vi "GOOPDebugger_AddDebugging.vi"(7 "Action":T1=enum."GeneratePattern", 8 "error in (no error)":errorcluster, 10 "DataIn":variant, 11 "ClassRefToActOn":refnum<vi>) -> (0 "error out":errorcluster, 1 "Name":string, 2 "DataOut":variant, 3 "Cancelled":bool)   [LabVIEW 2020]
uses:
  <resource>/Framework/Providers/Open_GDS/ClassProviders/Provider_BaseClassInterface/BaseProvider_SubVIs/BaseProvider_DesignPatternsActions.ctl
  <resource>/Framework/Providers/Open_GDS/ClassProviders/Common/LvClass_class/GDSLvClass_ProviderTypes.ctl
  <resource>/Framework/Providers/Open_GDS/ClassProviders/Provider_EndevoGOOP400/EndevoG4ProviderName.ctl
  <vilib>/picture/picture.llb/imagedata.ctl
panel:
  in  "_Cancel":bool
  in  "_OK":bool
  # "Debugging"
  # "This option will add debugging functions to the class"
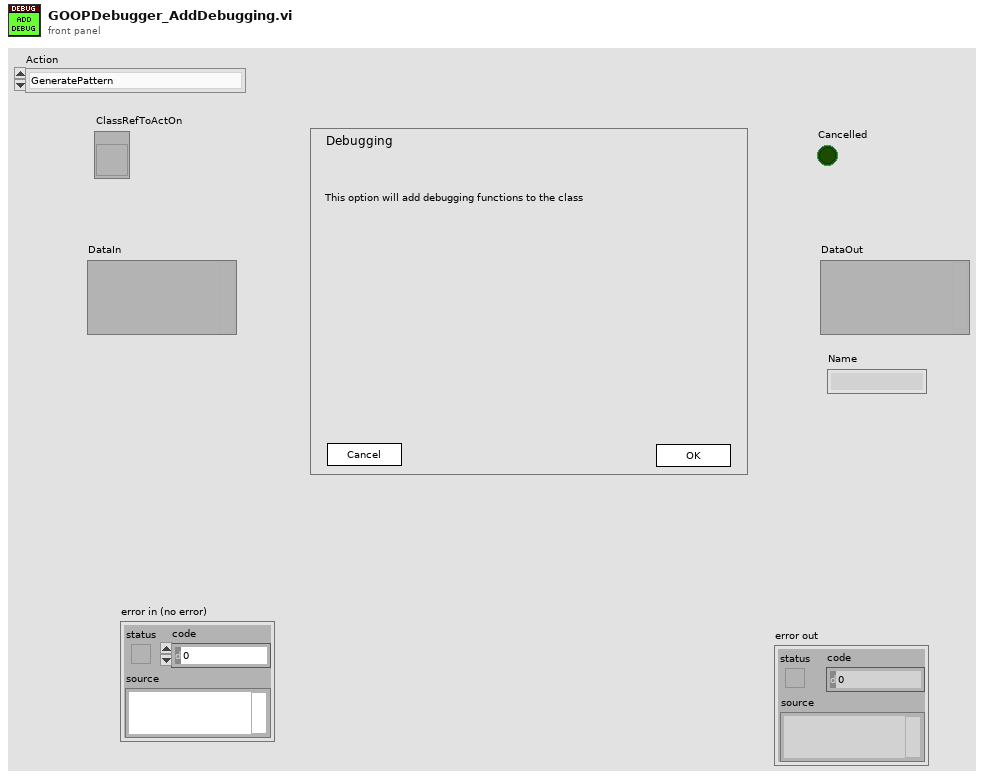
[diagram p1: front panel]
types:
  T1 = typedef "BaseProvider_DesignPatternsActions.ctl" = enum16{"AddPatternDialog", "GeneratePattern", "RemovePattern", "CreatePatternMethod", "UpdatePattern"}
  T2 = typedef "GDSLvClass_ProviderTypes.ctl" = enum16{"UnKnown(LabVOOP)", "Native", "EndevoGOOP3", "OpenG(RootObject)", "OpenG(OpenG_Object)", "EndevoGOOP4", "JKI1"}
  T3 = cluster{"Application":refnum<vi>, "SupportFolder":path, "TemplateName":string, "ClassProvider":T2, "UtilsFolder":path, "UtilsFolderRef":refnum<vi>, "ClassName":string, "Template_GetObjectStatus":path, "ProcessIdRef":refnum<vi>, "Template_GetObjectStatusRef":refnum<vi>, "ProtectedFolder":path, "ClassAttribute":bool}
  T4 = cluster{"Cancelled":bool, "Files":path[], "ClassPath":path, "DataOut":variant}
  T5 = typedef "EndevoG4ProviderName.ctl" = enum16{"EndevoGOOP400"}
  T6 = enum32{"invalid lock state", "Not Locked", "Locked (No Password)", "Password-protected"}
  T7 = typedef "imagedata.ctl" = cluster{"image type":i32, "image depth":i32, "image":u8[], "mask":u8[], "colors":u32[], "Rectangle":cluster{"left":i16, "top":i16, "right":i16, "bottom":i16}}
  T8 = typedef "GDSLvCLass_ClassSettingsType.ctl" = cluster{"ClassProviderName":string, "ClassTemplateUsed":string, "ClassTemplateVersion":string, "ClassDescription":string, "PlugIns":T9[], "ConnectorPanePattern":string}
  T9 = typedef "GDSLvClass_PlugIn.ctl" = cluster{"Type":T10, "ID":string, "Version":string, "Path":path, "Name":string, "Data":variant}
  T10 = typedef "GDSLvClass_PlugInTypes.ctl" = enum16{"DesignPattern", "MethodTypes"}
  T11 = typedef "GOOP400_Options.ctl" = cluster{"FlatFolderStructure":bool}
  T12 = typedef "GDSLvClass_IconSettingsType.ctl" = cluster{"Frame":u32, "Frame thickness":u8, "Header Background":u32, "Header Text":u32, "ColorPublic":u32, "ColorProtected":u32, "ColorPrivate":u32, "Body Text":u32, "ClassBodyIcon":string}
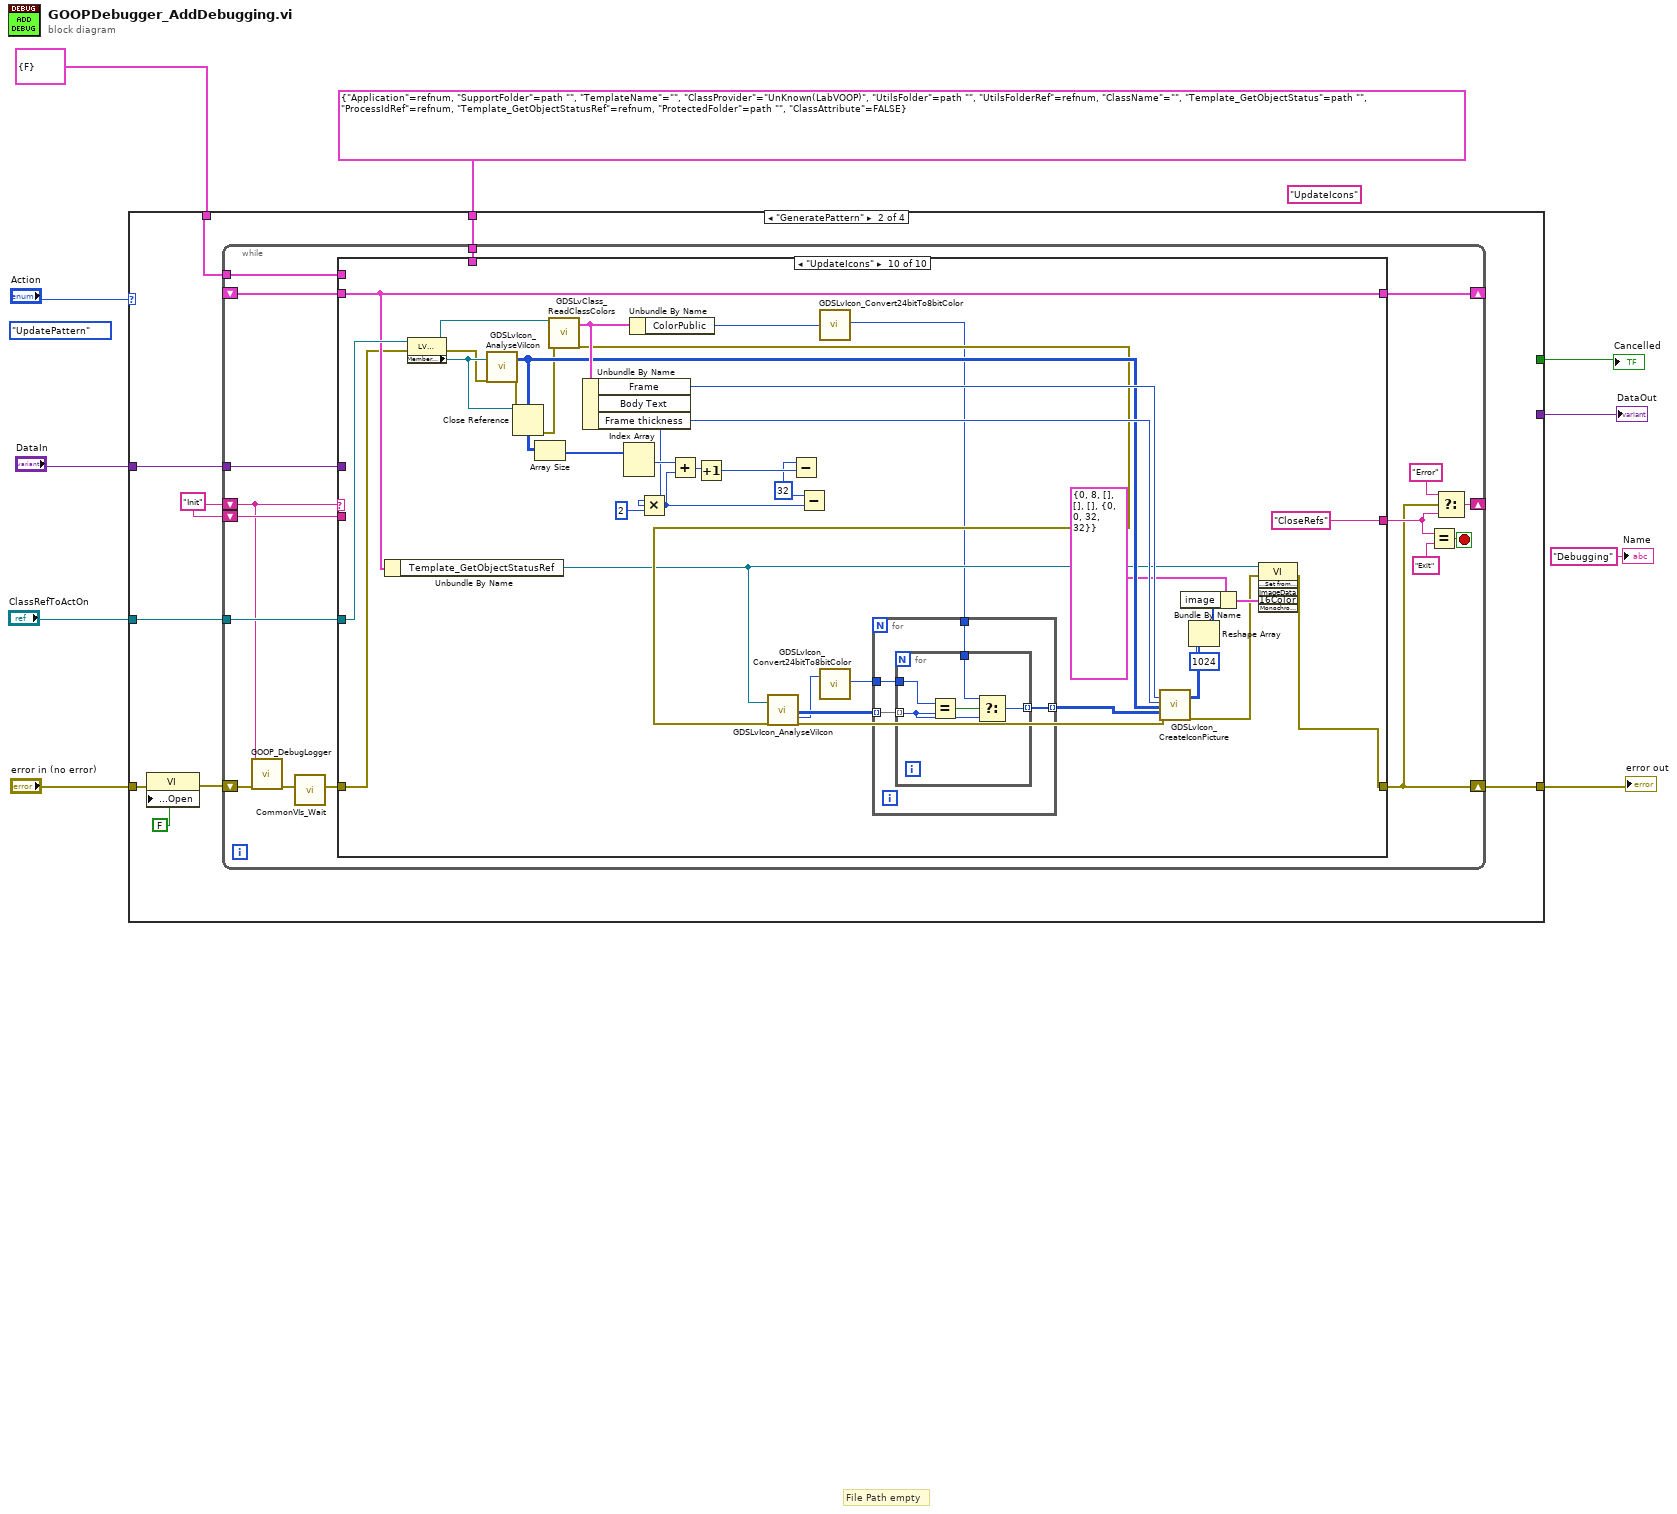
[diagram p0: block diagram]
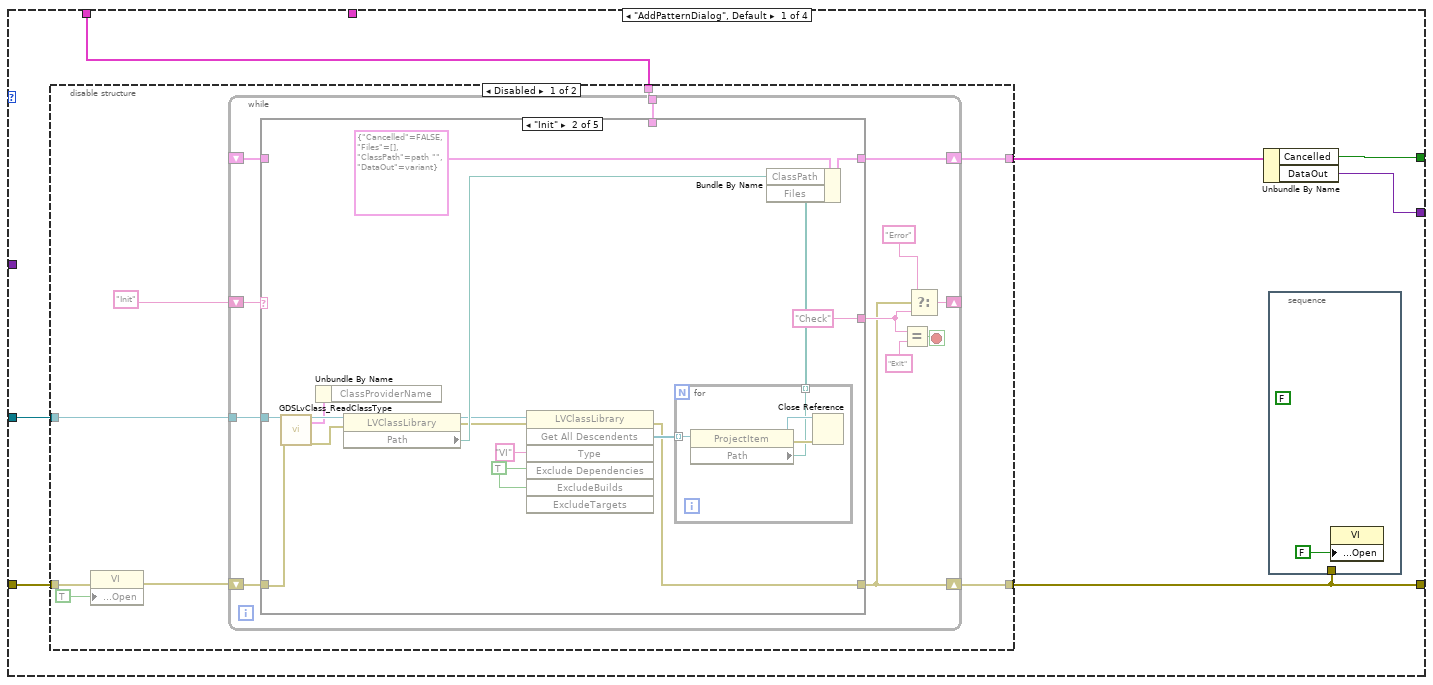
[diagram p2: hidden frame]
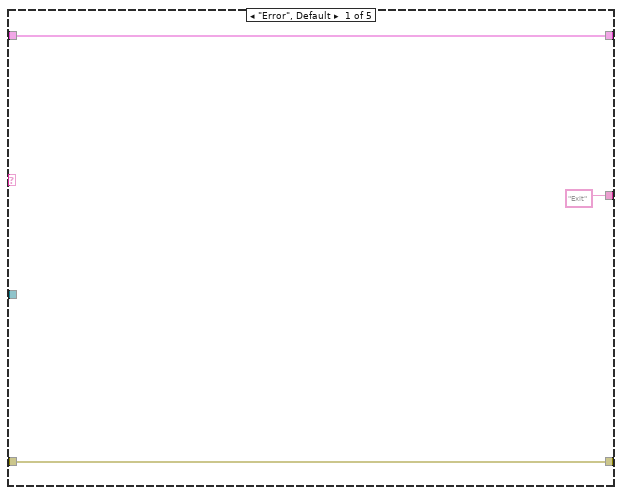
[diagram p3: hidden frame]
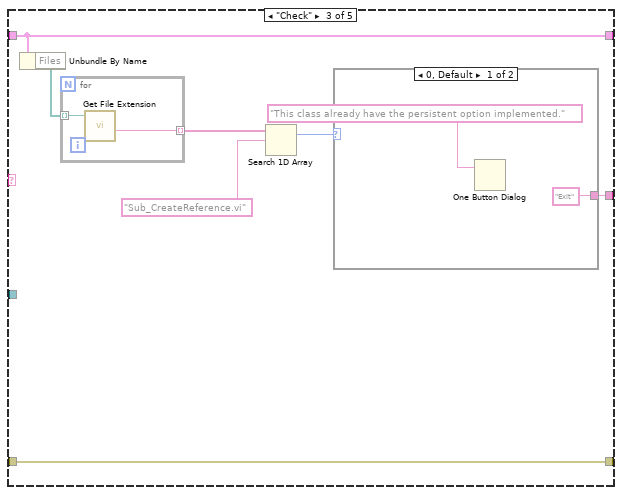
[diagram p4: hidden frame]
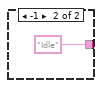
[diagram p5: hidden frame]
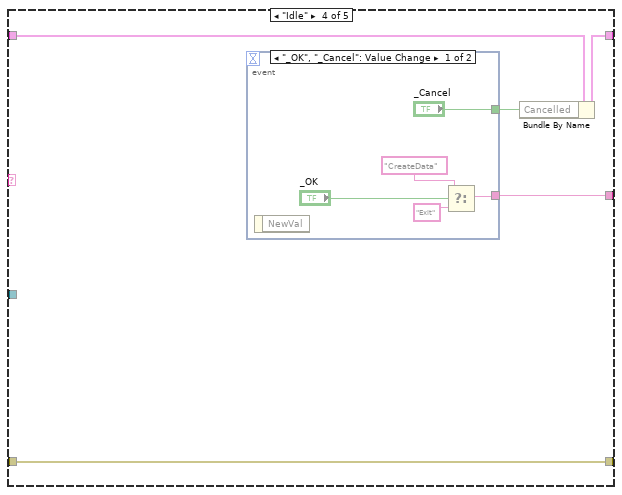
[diagram p6: hidden frame]
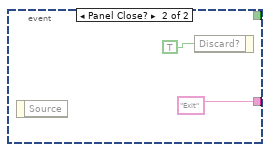
[diagram p7: hidden frame]
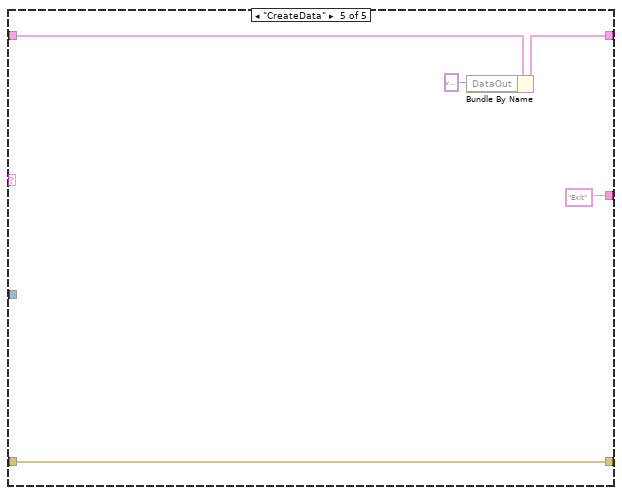
[diagram p8: hidden frame]
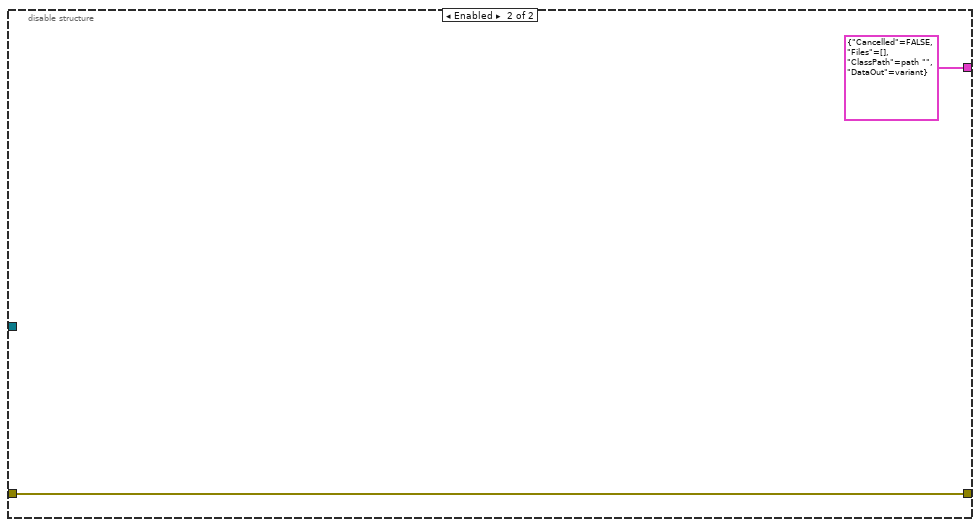
[diagram p9: hidden frame]
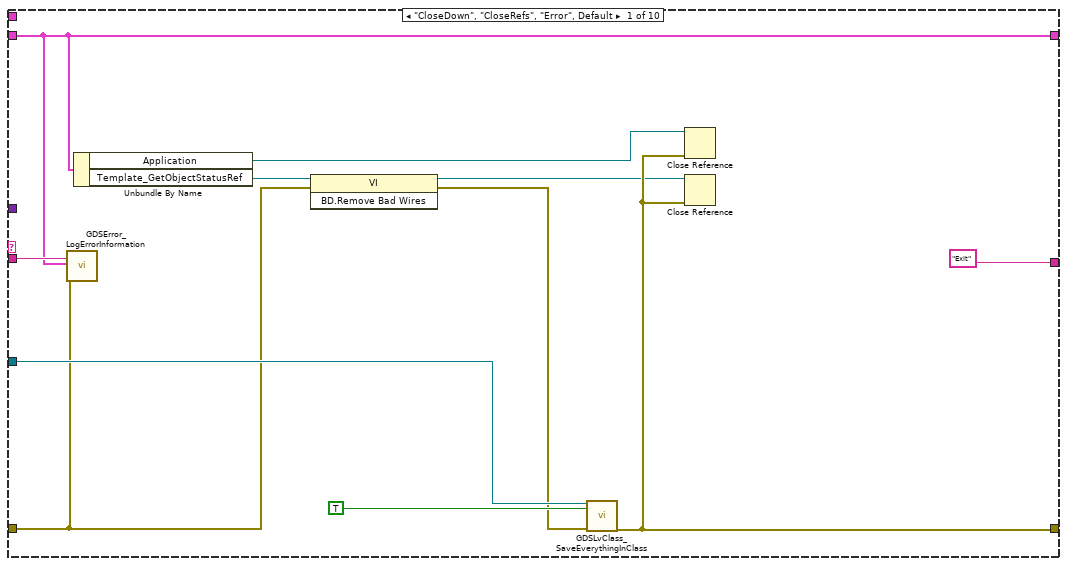
[diagram p10: hidden frame]
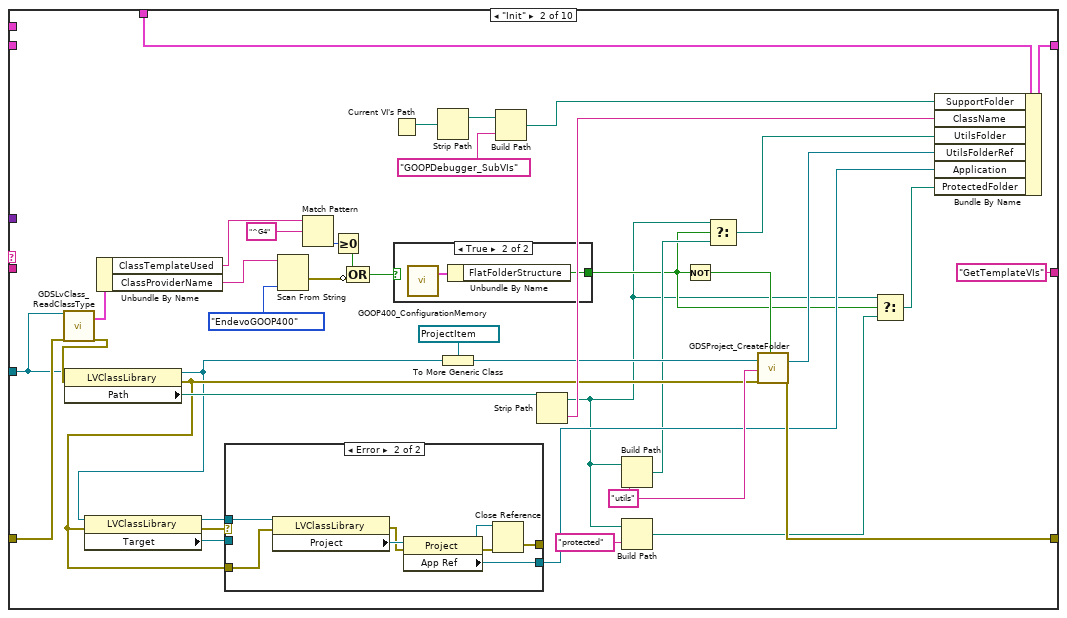
[diagram p11: hidden frame]
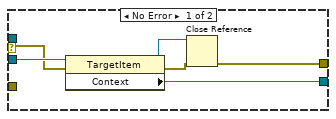
[diagram p13: hidden frame]
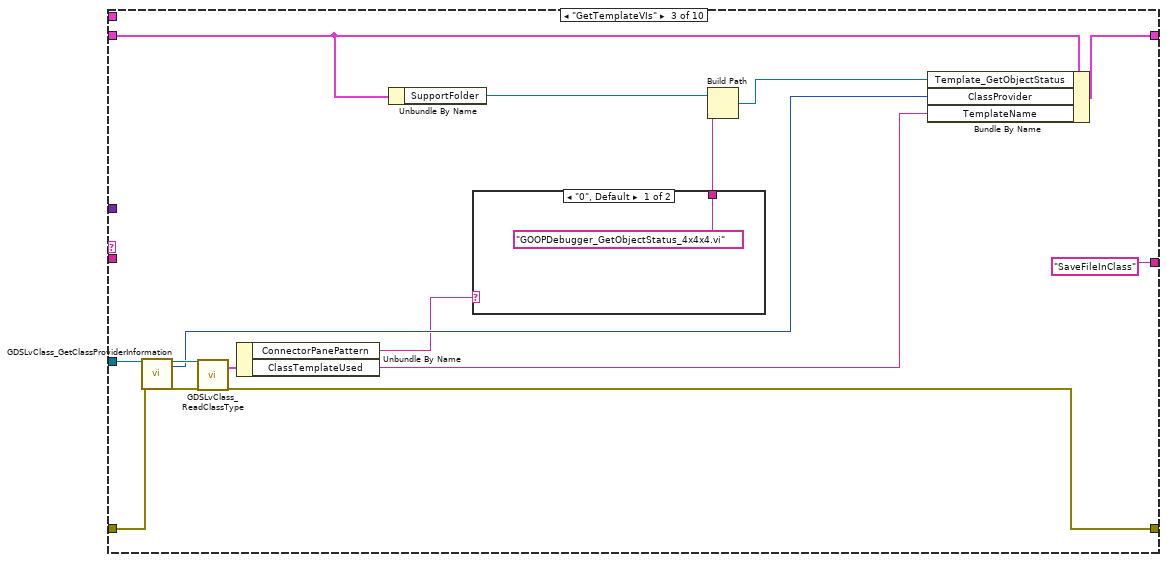
[diagram p14: hidden frame]
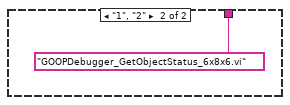
[diagram p15: hidden frame]
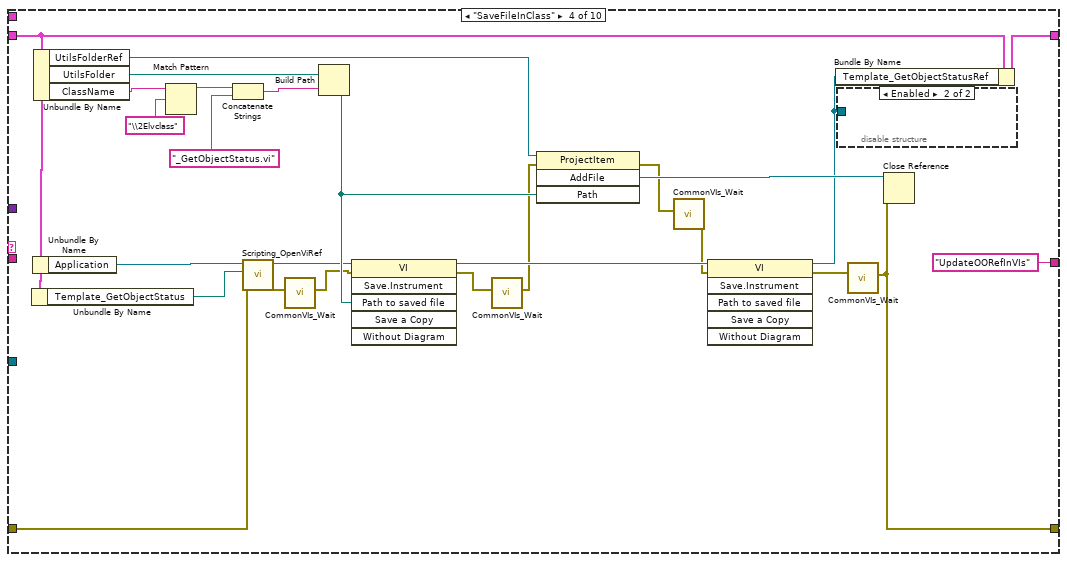
[diagram p16: hidden frame]
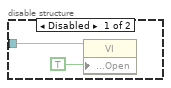
[diagram p17: hidden frame]
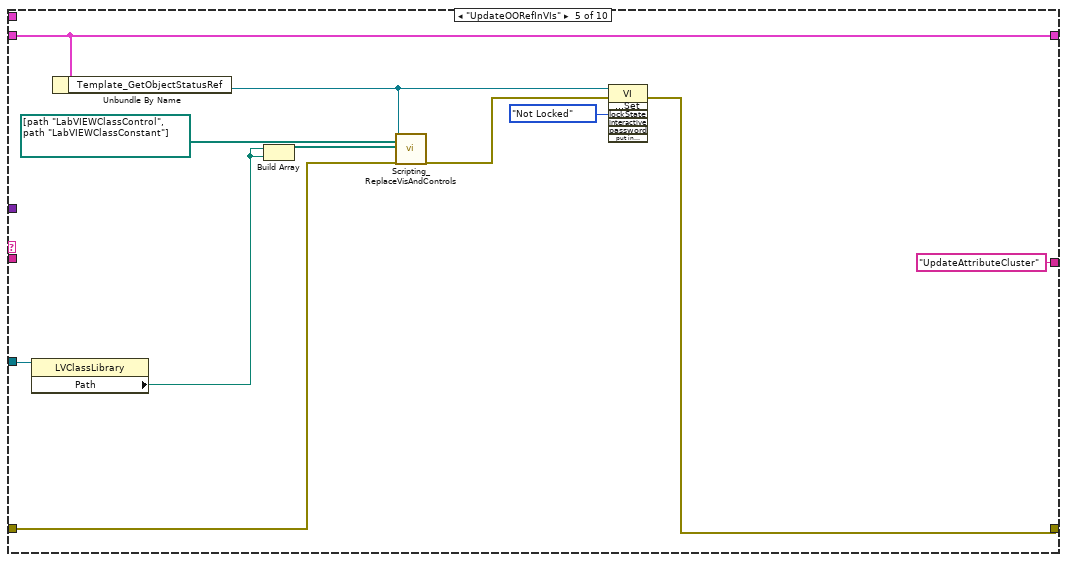
[diagram p18: hidden frame]
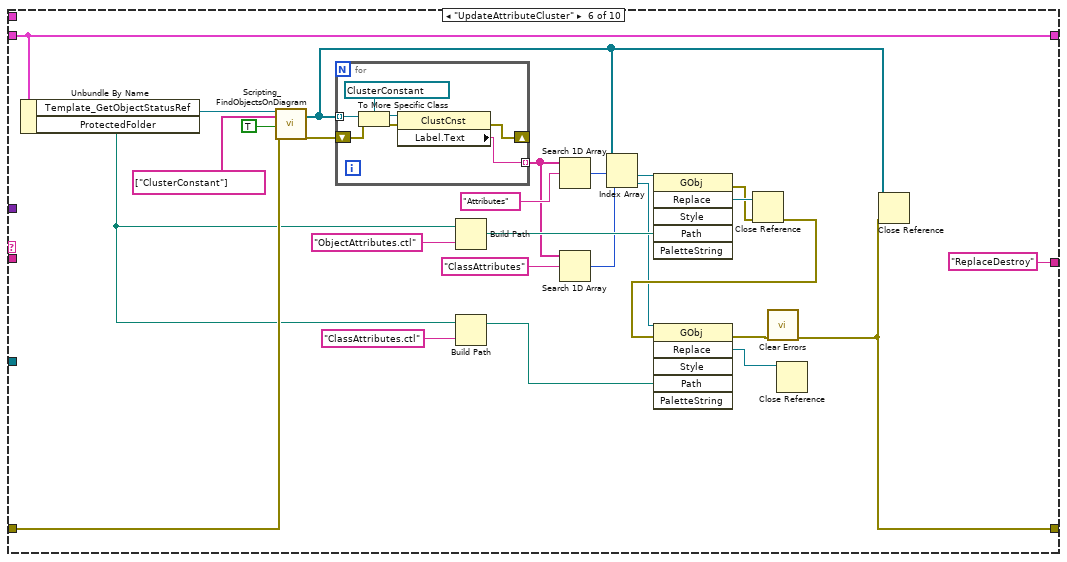
[diagram p19: hidden frame]
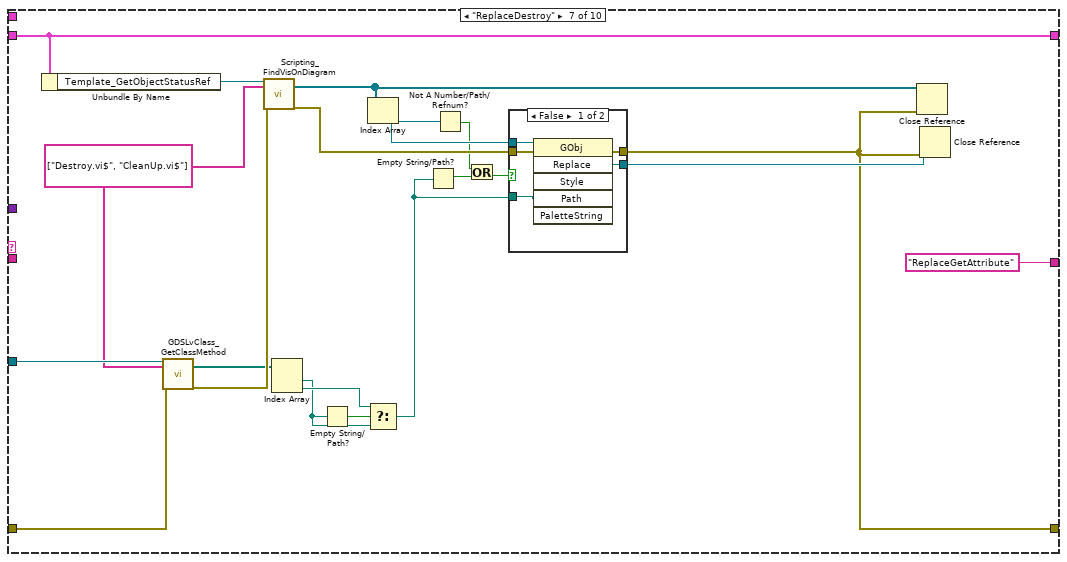
[diagram p20: hidden frame]
diagram:
  (unwired) "UpdateIcons"
  (unwired) BaseProvider_DesignPatternsActions."UpdatePattern" ("Action")
  # "File Path empty"
  n1 = case shown="\"GeneratePattern\"" "Action" {
    tunnel: "error in (no error)" -> [w17 w95 w421 w422]
    tunnel: [w16 w101 w421 w422] -> w8
    tunnel: "ClassRefToActOn" -> [w14 w97 _ _]
    tunnel: [w13 _ _ _] -> w6
    tunnel: [w12 _ _ _] -> w5
    tunnel: cluster{"Settings":bool} {"Settings"=FALSE} ("output cluster") -> [w11 w99 _ _]
    tunnel: "DataIn" -> [_ w100 _ _]
    tunnel: T3 {"Application"=refnum, "SupportFolder"=path "", "TemplateName"="", "ClassProvider"=enum."UnKnown(LabVOOP)", "UtilsFolder"=path "", "UtilsFolderRef"=refnum, "ClassName"="", "Template_GetObjectStatus"=path "", "ProcessIdRef"=refnum, "Template_GetObjectStatusRef"=refnum, "ProtectedFolder"=path "", "ClassAttribute"=FALSE} -> [_ w98 _ _]
    frame "AddPatternDialog", Default {
      n2 = disable-structure shown="Disabled" {
        disable-tunnel: w17 -> [w24 w91]
        disable-tunnel: [w21 w91] -> w16
        disable-tunnel: [w20 T4 {"Cancelled"=FALSE, "Files"=[], "ClassPath"=path "", "DataOut"=variant}] -> w15
        disable-tunnel: w14 -> [w19 _]
        disable-tunnel: w11 -> [w18 _]
        frame Disabled {
          n3 = property class="VI"(error in=w24, "Front Panel.Open"=TRUE ("Front Panel Window:Open")) -> (error out=w23:errorcluster)  [unwired: 1 in, 1 out]
          n4 = while {
            shift-right: [w30] -> w21
            shift-left: w23 -> [w37]
            shift-right: [w35] -> _
            shift-left: "Init" -> [w36]
            shift-right: [w29] -> w20
            shift-left: _ -> [w28]
            tunnel: w19 -> [w27]
            tunnel: w18 -> [w26]
            stop <- w34 stop-if-true
            n5 = case shown="\"Init\"" w36 {
              tunnel: w37 -> [w40 w43 w64 w76 w86]
              tunnel: [w40 w52 w64 w76 w86] -> w30
              tunnel: ["Exit" "Check" w66 w77 "Exit"] -> w31
              tunnel: [w38 w50 w65 w75 w88] -> w29
              tunnel: w28 -> [w38 _ w65 w73 w89]
              tunnel: w27 -> [_ w45 _ _ _]
              tunnel: w26 -> [_ _ _ _ _]
              frame "Error", Default {
              }
              frame "Init" {
                w54 = TRUE ("ExcludeDependencies")
                n6 = call <resource>:"GDSLvClass_ReadClassType.vi"("Class Refnum In"=w45, "error in (no error)"=w43) -> ("Class Refnum Out"=w44:refnum<vi>, "ClassSettings"=w41:T8, "error out"=w42:errorcluster)  [unwired: 15 in]
                n7 = Unbundle By Name(w41) -> ()  [unwired: 1 out]
                n8 = property class="LVClassLibrary"(reference=w44, error in=w42) -> (reference out=w47:refnum<vi>, error out=w46:errorcluster, "Path"=w49:path)
                n9 = invoke class="LVClassLibrary" method="Get All Descendents"(reference=w47, error in=w46, "Type"="VI", "Exclude Dependencies"=w54, "ExcludeBuilds"=w54) -> (error out=w52:errorcluster, "All Descendents"=w53:refnum<vi>[])  [unwired: 2 in, 5 out]
                n10 = for {
                  tunnel: w53 -> [w60] mode=indexing
                  tunnel: [w57] -> w48 mode=indexing
                  n11 = property class="ProjectItem"(reference=w60) -> (reference out=w58:refnum<vi>, error out=w59:errorcluster, "Path"=w57:path)  [unwired: 1 in]
                  n12 = Close Reference(reference=w58, error in (no error)=w59) -> ()  [unwired: 1 out]
                }
                n13 = Bundle By Name(cluster=T4 {"Cancelled"=FALSE, "Files"=[], "ClassPath"=path "", "DataOut"=variant}, "ClassPath"=w49, "Files"=w48) -> (w50:T4)
              }
              frame "Check" {
                n14 = Unbundle By Name(w65) -> ("Files"=w67:path[])
                n15 = for {
                  tunnel: w67 -> [w72] mode=indexing
                  tunnel: [w71] -> w63 mode=indexing
                  n16 = call <vilib>:"Get File Extension.vi"("file"=w72) -> ("filename without extension"=w71:string)  [unwired: 6 in, 4 out]
                }
                n17 = Search 1D Array(1D array=w63, element="Sub_CreateReference.vi") -> (index of element=w61:i32)  [unwired: 1 in]
                n18 = case shown="0, Default" w61 {
                  tunnel: ["Exit" "Idle"] -> w66
                  frame 0, Default {
                    n19 = One Button Dialog(message="This class already have the persistent option implemented.") -> ()  [unwired: 1 in, 1 out]
                  }
                  frame -1 {
                  }
                }
              }
              frame "Idle" {
                n20 = event shown="[0] \"_OK\", \"_Cancel\": Value Change" {
                  selector: _ -> [_ _]
                  dyn-events: _ -> [_ _]
                  timeout: _ -> [_ _]
                  tunnel: [w81 "Exit"] -> w77
                  tunnel: ["_Cancel" _] -> w74
                  event "_OK", "_Cancel": Value Change {
                    n21 = event-data() -> ()  [unwired: 1 in, 1 out]
                    n22 = Select(t="CreateData", s="_OK", f="Exit") -> (s? t:f=w81:string)
                  }
                  event Panel Close? {
                    n23 = event-data() -> ()  [unwired: 1 in, 1 out]
                    n24 = event-data("Discard?"=TRUE) -> ()  [unwired: 1 in, 1 out]
                  }
                }
                n25 = Bundle By Name(cluster=w73, "Cancelled"=w74) -> (w75:T4)
              }
              frame "CreateData" {
                n26 = Bundle By Name(cluster=w89, "DataOut"=variant) -> (w88:T4)
              }
            }
            n27 = Equal?(x=w31, y="Exit") -> (x = y?=w34:bool)
            n28 = Select(t="Error", s=w30, f=w31) -> (s? t:f=w35:string)
          }
        }
        frame Enabled {
        }
      }
      n29 = Unbundle By Name(w15) -> ("Cancelled"=w13:bool, "DataOut"=w12:variant)
      n30 = stacked-sequence {
        tunnel: w16 -> [_]
        frame #0 {
          (unwired) FALSE ("Visible")
          n31 = property class="VI"("Front Panel.Open"=FALSE ("Front Panel Window:Open")) -> ()  [unwired: 2 in, 2 out]
        }
      }
    }
    frame "GeneratePattern" {
      w93 = "Init"
      n32 = property class="VI"(error in=w95, "Front Panel.Open"=FALSE ("Front Panel Window:Open")) -> (error out=w94:errorcluster)  [unwired: 1 in, 1 out]
      n33 = while {
        shift-right: [w113] -> w101
        shift-left: w94 -> [w105]
        shift-right: [w118] -> _
        shift-left: w93 -> [w104]
        shift-right: [w112] -> _
        shift-left: _ -> [w111]
        tunnel: w100 -> [w110]
        tunnel: w99 -> [w109]
        tunnel: w98 -> [w108]
        tunnel: w97 -> [w107]
        shift-left: w93 -> [w106]
        stop <- w117 stop-if-true
        n34 = call <resource>:"GOOP_DebugLogger.vi"("error in (no error)"=w105, "State"=w104) -> ("error out"=w103:errorcluster)  [unwired: 7 in, 2 out]
        n35 = call <resource>:"CommonVIs_Wait.vi"("error in"=w103) -> ("error out"=w102:errorcluster)  [unwired: 9 in]
        n36 = case shown="\"UpdateIcons\"" w104 {
          tunnel: w102 -> [w120 w139 w199 w222 w240 w257 w288 w321 w362 w391]
          tunnel: [w125 w161 w188 w203 w234 w245 w275 w322 w361 w390] -> w113
          tunnel: ["Exit" "GetTemplateVIs" "SaveFileInClass" "UpdateOORefInVIs" "UpdateAttributeCluster" "ReplaceDestroy" "ReplaceGetAttribute" w311 "UpdateIcons" "CloseRefs"] -> w114
          tunnel: [w123 w168 w198 w228 w241 w242 w285 w309 w360 w393] -> w112
          tunnel: w111 -> [w123 _ w193 w226 w241 w242 w285 w310 w360 w393]
          tunnel: w110 -> [_ _ _ _ _ _ _ _ _ _]
          tunnel: w109 -> [_ _ _ _ _ _ _ _ _ _]
          tunnel: w108 -> [_ w167 _ _ _ _ _ _ _ _]
          tunnel: w107 -> [w127 w138 w200 _ w239 _ w290 w318 _ w394]
          tunnel: w106 -> [w124 _ _ _ _ _ _ _ _ _]
          frame "CloseDown", "CloseRefs", "Error", Default {
            n37 = call <resource>:"GDSError_LogErrorInformation.vi"("State"=w124, "LocalVariableData"=w123, "error in (no error)"=w120) -> ()  [unwired: 16 in, 1 out]
            n38 = Unbundle By Name(w123) -> ("Application"=w126:refnum<vi>, "Template_GetObjectStatusRef"=w122:refnum<vi>)
            n39 = invoke class="VI" method="BD.Remove Bad Wires"(reference=w122, error in=w120) -> (reference out=w121:refnum<vi>, error out=w119:errorcluster)  [unwired: 1 in, 1 out]
            n40 = call <resource>:"GDSLvClass_SaveEverythingInClass.vi"("ClassRefIn"=w127, "ForceResaving(False)"=TRUE, "error in"=w119) -> ("error out"=w125:errorcluster)  [unwired: 15 in, 1 out]
            n41 = Close Reference(reference=w126, error in (no error)=w125) -> ()  [unwired: 1 out]
            n42 = Close Reference(reference=w121, error in (no error)=w125) -> ()  [unwired: 1 out]
          }
          frame "Init" {
            w157 = "utils" ("name or relative path")
            n43 = call <resource>:"GDSLvClass_ReadClassType.vi"("Class Refnum In"=w138, "error in (no error)"=w139) -> ("ClassSettings"=w143:T8, "error out"=w140:errorcluster)  [unwired: 15 in, 1 out]
            n44 = property class="LVClassLibrary"(reference=w138, error in=w140) -> (reference out=w130:refnum<vi>, error out=w150:errorcluster, "Path"=w162:path)
            n45 = property class="LVClassLibrary"(reference=w130, error in=w150) -> (reference out=w152:refnum<vi>, error out=w154:errorcluster, "Target"=w153:refnum<vi>)
            n46 = Unbundle By Name(w143) -> ("ClassTemplateUsed"=w142:string, "ClassProviderName"=w141:string)
            n47 = case shown="Error" w154 {
              selector: w154 -> [w173 _]
              tunnel: w153 -> [w177 _]
              tunnel: [w176 w179] -> w151
              tunnel: [w172 w180] -> _
              tunnel: w152 -> [_ w185]
              tunnel: w150 -> [_ w184]
              frame No Error {
                n48 = property class="TargetItem"(reference=w177, error in=w173) -> (reference out=w174:refnum<vi>, error out=w175:errorcluster, "Context"=w176:refnum<vi>)
                n49 = Close Reference(reference=w174, error in (no error)=w175) -> (error out=w172:errorcluster)
              }
              frame Error {
                n50 = property class="LVClassLibrary"(reference=w185, error in=w184) -> (error out=w178:errorcluster, "Project"=w183:refnum<vi>)  [unwired: 1 out]
                n51 = property class="Project"(reference=w183, error in=w178) -> (reference out=w181:refnum<vi>, error out=w182:errorcluster, "App Ref"=w179:refnum<vi>)
                n52 = Close Reference(reference=w181, error in (no error)=w182) -> (error out=w180:errorcluster)
              }
            }
            n53 = Scan From String(input string=w141, default 1=EndevoG4ProviderName."EndevoGOOP400" ("ProviderName")) -> (error out=w147:errorcluster)  [unwired: 4 in, 2 out]
            n54 = Match Pattern(string=w142, regular expression="^G4") -> (offset past match=w146:i32)  [unwired: 1 in, 3 out]
            n55 = Greater Or Equal To 0?(x=w146) -> (x >= 0?=w148:bool)
            n56 = Compound Arithmetic op=OR(w148, invert w147) -> (w149:bool)
            n57 = Current VI's Path() -> (path=w165:path)
            n58 = case shown="True" w149 {
              tunnel: [_ w170] -> w134
              frame False {
              }
              frame True {
                n59 = call <resource>:"GOOP400_ConfigurationMemory.vi"() -> ("OptionsOut"=w171:T11)  [unwired: 18 in, 1 out]
                n60 = Unbundle By Name(w171) -> ("FlatFolderStructure"=w170:bool)
              }
            }
            n61 = Strip Path(path=w165) -> (stripped path=w164:path)  [unwired: 1 out]
            n62 = To More Generic Class(target class=refnum<vi> refnum ("AddItem"), reference=w130) -> (generic class reference=w156:refnum<vi>)
            n63 = Build Path(base path=w164, name or relative path="GOOPDebugger_SubVIs") -> (appended path=w160:path)
            n64 = Strip Path(path=w162) -> (stripped path=w133:path, name=w158:string)
            n65 = Build Path(base path=w133, name or relative path=w157) -> (appended path=w136:path)
            n66 = Build Path(base path=w133, name or relative path="protected") -> (appended path=w132:path)
            n67 = Not(x=w134) -> (.not. x?=w137:bool)
            n68 = Select(t=w133, s=w134, f=w136) -> (s? t:f=w135:path)
            n69 = call <resource>:"GDSProject_CreateFolder.vi"("Project Item To Create Folder Below(Use MyComputer if not wired)"=w156, "FolderName"=w157, "error in (no error)"=w150, "CreateThePhysicalFolderIfPossible(False)"=w137) -> ("ItemOut"=w159:refnum<vi>, "error out"=w161:errorcluster)  [unwired: 12 in, 2 out]
            n70 = Select(t=w133, s=w134, f=w132) -> (s? t:f=w131:path)
            n71 = Bundle By Name(cluster=w167, "SupportFolder"=w160, "ClassName"=w158, "UtilsFolder"=w135, "UtilsFolderRef"=w159, "Application"=w151, "ProtectedFolder"=w131) -> (w168:T3)
          }
          frame "GetTemplateVIs" {
            n72 = call <resource>:"GDSLvClass_GetClassProviderInformation.vi"("Class Refnum In"=w200, "error in (no error)"=w199) -> ("Class Refnum Out"=w197:refnum<vi>, "ClassProvider"=w189:T2, "error out"=w196:errorcluster)  [unwired: 15 in]
            n73 = call <resource>:"GDSLvClass_ReadClassType.vi"("Class Refnum In"=w197, "error in (no error)"=w196) -> ("ClassSettings"=w192:T8, "error out"=w188:errorcluster)  [unwired: 15 in, 1 out]
            n74 = Unbundle By Name(w192) -> ("ConnectorPanePattern"=w186:string, "ClassTemplateUsed"=w187:string)
            n75 = Unbundle By Name(w193) -> ("SupportFolder"=w195:path)
            n76 = case shown="\"0\", Default" w186 {
              tunnel: ["GOOPDebugger_GetObjectStatus_4x4x4.vi" ("name or relative path") "GOOPDebugger_GetObjectStatus_6x8x6.vi" ("name or relative path")] -> w194
              frame "0", Default {
              }
              frame "1", "2" {
              }
            }
            n77 = Build Path(base path=w195, name or relative path=w194) -> (appended path=w190:path)
            n78 = Bundle By Name(cluster=w193, "Template_GetObjectStatus"=w190, "ClassProvider"=w189, "TemplateName"=w187) -> (w198:T3)
          }
          frame "SaveFileInClass" {
            n79 = Unbundle By Name(w226) -> ("Template_GetObjectStatus"=w221:path)
            n80 = Unbundle By Name(w226) -> ("Application"=w220:refnum<vi>)
            n81 = Unbundle By Name(w226) -> ("UtilsFolderRef"=w216:refnum<vi>, "UtilsFolder"=w212:path, "ClassName"=w225:string)
            n82 = Match Pattern(string=w225, regular expression="\\2Elvclass") -> (before substring=w219:string)  [unwired: 1 in, 3 out]
            n83 = Concatenate Strings(w219, "_GetObjectStatus.vi" ("name or relative path")) -> (w217:string)
            n84 = call <resource>:"Scripting_OpenViRef.vi"("error in"=w222, "ViPath/ViName/Viref"=w221, "AppRef"=w220) -> ("error out"=w208:errorcluster, "vi reference"=w213:refnum<vi>)  [unwired: 6 in, 1 out]
            n85 = call <resource>:"CommonVIs_Wait.vi"("error in"=w208) -> ("error out"=w207:errorcluster)  [unwired: 9 in]
            n86 = Build Path(base path=w212, name or relative path=w217) -> (appended path=w214:path)
            n87 = invoke class="VI" method="Save.Instrument"(reference=w213, error in=w207, "Path to saved file"=w214) -> (reference out=w215:refnum<vi>, error out=w206:errorcluster)  [unwired: 3 in, 4 out]
            n88 = call <resource>:"CommonVIs_Wait.vi"("error in"=w206) -> ("error out"=w205:errorcluster)  [unwired: 9 in]
            n89 = invoke class="ProjectItem" method="AddFile"(reference=w216, error in=w205, "Path"=w214) -> (error out=w210:errorcluster, "AddFile"=w223:refnum<vi>)  [unwired: 1 in, 2 out]
            n90 = call <resource>:"CommonVIs_Wait.vi"("error in"=w210) -> ("error out"=w209:errorcluster)  [unwired: 9 in]
            n91 = invoke class="VI" method="Save.Instrument"(reference=w215, error in=w209) -> (reference out=w211:refnum<vi>, error out=w204:errorcluster)  [unwired: 4 in, 4 out]
            n92 = Bundle By Name(cluster=w226, "Template_GetObjectStatusRef"=w211) -> (w228:T3)
            n93 = disable-structure shown="Enabled" {
              disable-tunnel: w211 -> [w230 _]
              frame Disabled {
                n94 = property class="VI"(reference=w230, "Front Panel.Open"=TRUE ("Front Panel Window:Open")) -> ()  [unwired: 1 in, 2 out]
              }
              frame Enabled {
              }
            }
            n95 = call <resource>:"CommonVIs_Wait.vi"("error in"=w204) -> ("error out"=w203:errorcluster)  [unwired: 9 in]
            n96 = Close Reference(reference=w223, error in (no error)=w203) -> ()  [unwired: 1 out]
          }
          frame "UpdateOORefInVIs" {
            n97 = property class="LVClassLibrary"(reference=w239) -> ("Path"=w235:path)  [unwired: 1 in, 2 out]
            n98 = Unbundle By Name(w241) -> ("Template_GetObjectStatusRef"=w231:refnum<vi>)
            n99 = Build Array(w235, w235) -> (w233:path[])
            n100 = call <resource>:"Scripting_ReplaceVisAndControls.vi"("ViRef"=w231, "OldVIsAndControls"=path[] [path "LabVIEWClassControl", path "LabVIEWClassConstant"], "NewVIsAndControls"=w233, "error in (no error)"=w240) -> ("error out"=w236:errorcluster)  [unwired: 15 out]
            n101 = invoke class="VI" method="Lock State.Set"(reference=w231, error in=w236, "lockState"=T6."Not Locked" ("Lock State")) -> (error out=w234:errorcluster)  [unwired: 4 in, 6 out]
          }
          frame "UpdateAttributeCluster" {
            n102 = Unbundle By Name(w242) -> ("Template_GetObjectStatusRef"=w266:refnum<vi>, "ProtectedFolder"=w250:path)
            n103 = call <resource>:"Scripting_FindObjectsOnDiagram.vi"("ViRef(Ignored If Not Wired)"=w266, "NodeTypesToSearchFor"=string[] ["ClusterConstant"], "Don'tSearchSubStructures(False)"=TRUE, "error in (no error)"=w257) -> ("Nodes"=w252:refnum<vi>[], "error out"=w263:errorcluster)  [unwired: 14 in]
            n104 = for {
              tunnel: w252 -> [w273] mode=indexing
              shift-right: [w269] -> _
              shift-left: w263 -> [w270]
              tunnel: [w268] -> w256 mode=indexing
              n105 = To More Specific Class(target class=refnum<vi> refnum ("WhileLoop"), reference=w273, error in=w270) -> (specific class reference=w272:refnum<vi>, error out=w271:errorcluster)
              n106 = property class="ClustCnst"(reference=w272, error in=w271) -> (error out=w269:errorcluster, "Label.Text"=w268:string)  [unwired: 1 out]
            }
            n107 = Build Path(base path=w250, name or relative path="ObjectAttributes.ctl") -> (appended path=w260:path)
            n108 = Build Path(base path=w250, name or relative path="ClassAttributes.ctl") -> (appended path=w248:path)
            n109 = Search 1D Array(1D array=w256, element="Attributes") -> (index of element=w254:i32)  [unwired: 1 in]
            n110 = Search 1D Array(1D array=w256, element="ClassAttributes") -> (index of element=w243:i32)  [unwired: 1 in]
            n111 = Index Array(array=w252, index #1=w254, index #2=w243) -> (element #1=w253:refnum<vi>, element #2=w244:refnum<vi>)
            n112 = invoke class="GObj" method="Replace"(reference=w253, "Path"=w260) -> (error out=w258:errorcluster, "Replace"=w259:refnum<vi>)  [unwired: 4 in, 4 out]
            n113 = Close Reference(reference=w259, error in (no error)=w258) -> (error out=w249:errorcluster)
            n114 = invoke class="GObj" method="Replace"(reference=w244, error in=w249, "Path"=w248) -> (error out=w247:errorcluster, "Replace"=w246:refnum<vi>)  [unwired: 3 in, 4 out]
            n115 = call <vilib>:"Clear Errors.vi"("error in (no error)"=w247) -> ("error out"=w245:errorcluster)  [unwired: 5 in, 1 out]
            n116 = Close Reference(reference=w246) -> ()  [unwired: 1 in, 1 out]
            n117 = Close Reference(reference=w252, error in (no error)=w245) -> ()  [unwired: 1 out]
          }
          frame "ReplaceDestroy" {
            w289 = string[] ["Destroy.vi$", "CleanUp.vi$"] ("VIsToSerachFor/ViName")
            n118 = Unbundle By Name(w285) -> ("Template_GetObjectStatusRef"=w276:refnum<vi>)
            n119 = call <resource>:"GDSLvClass_GetClassMethod.vi"("Class Refnum In"=w290, "VINames"=w289, "error in (no error)"=w288) -> ("ViPaths"=w286:path[], "error out"=w287:errorcluster)  [unwired: 13 in, 2 out]
            n120 = call <resource>:"Scripting_FindVisOnDiagram.vi"("ViRef"=w276, "VIsToSerachFor/ViName"=w289, "error in (no error)"=w287) -> ("VisFound"=w292:refnum<vi>[], "error out"=w291:errorcluster)  [unwired: 15 in]
            n121 = Index Array(array=w286) -> (element #1=w282:path, element #2=w283:path)  [unwired: 2 in]
            n122 = Empty String/Path?(string/path=w282) -> (empty?=w284:bool)
            n123 = Index Array(array=w292) -> (element=w280:refnum<vi>)  [unwired: 1 in]
            n124 = Select(t=w283, s=w284, f=w282) -> (s? t:f=w281:path)
            n125 = Empty String/Path?(string/path=w281) -> (empty?=w279:bool)
            n126 = Not A Number/Path/Refnum?(number/path/refnum=w280) -> (NaN/Path/Refnum?=w278:bool)
            n127 = Or(x=w278, y=w279) -> (x .or. y?=w277:bool)
            n128 = case shown="False" w277 {
              tunnel: [w299 _] -> w293
              tunnel: w291 -> [w298 w300]
              tunnel: [w297 w300] -> w275
              tunnel: w281 -> [w296 _]
              tunnel: w280 -> [w295 _]
              frame False {
                n129 = invoke class="GObj" method="Replace"(reference=w295, error in=w298, "Path"=w296) -> (error out=w297:errorcluster, "Replace"=w299:refnum<vi>)  [unwired: 3 in, 4 out]
              }
              frame True {
              }
            }
            n130 = Close Reference(reference=w292, error in (no error)=w275) -> ()  [unwired: 1 out]
            n131 = Close Reference(reference=w293, error in (no error)=w275) -> ()  [unwired: 1 out]
          }
          frame "ReplaceGetAttribute" {
            w331 = string[] ["_GetAttributes.vi$"] ("VIsToSerachFor/ViName")
            n132 = Unbundle By Name(w310) -> ("Template_GetObjectStatusRef"=w324:refnum<vi>)
            n133 = call <resource>:"GDSLvClass_GetClassMethod.vi"("Class Refnum In"=w318, "VINames"=string[] ["_GetClassAttributes.vi"] ("VIsToSerachFor/ViName"), "error in (no error)"=w321) -> ("ViPaths"=w314:path[], "error out"=w320:errorcluster)  [unwired: 13 in, 2 out]
            n134 = call <resource>:"GDSLvClass_GetClassMethod.vi"("Class Refnum In"=w318, "VINames"=w331, "error in (no error)"=w320) -> ("ViPaths"=w329:path[], "error out"=w330:errorcluster)  [unwired: 13 in, 2 out]
            n135 = call <resource>:"Scripting_FindVisOnDiagram.vi"("ViRef"=w324, "VIsToSerachFor/ViName"=w331, "error in (no error)"=w330) -> ("VisFound"=w304:refnum<vi>[], "error out"=w306:errorcluster)  [unwired: 15 in]
            n136 = for {
              shift-right: [w334] -> w305
              shift-left: w306 -> [w338]
              tunnel: w304 -> [w339] mode=indexing
              tunnel: [w333] -> w302 mode=indexing
              w337 = refnum<vi> refnum  # SubVI
              n137 = To More Specific Class(target class=w337, reference=w339, error in=w338) -> (specific class reference=w336:refnum<vi>, error out=w335:errorcluster)
              n138 = property class="SubVI"(reference=w336, error in=w335) -> (error out=w334:errorcluster, "VI Ref"=w333:refnum<vi>)  [unwired: 1 out]
            }
            n139 = Index Array(array=w314) -> (element #1=w317:path, element #2=w316:path)  [unwired: 2 in]
            n140 = Index Array(array=w329) -> (element #1=w326:path, element #2=w327:path)  [unwired: 2 in]
            n141 = Empty String/Path?(string/path=w317) -> (empty?=w315:bool)
            n142 = Empty String/Path?(string/path=w326) -> (empty?=w328:bool)
            n143 = Select(t=w316, s=w315, f=w317) -> (s? t:f=w307:path)
            n144 = Select(t=w327, s=w328, f=w326) -> (s? t:f=w325:path)
            n145 = Empty String/Path?(string/path=w307) -> (empty?=w308:bool)
            n146 = for {
              tunnel: [w343] -> w332 mode=indexing
              tunnel: w325 -> [w357]
              shift-right: [w341] -> w323
              shift-left: w305 -> [w355]
              tunnel: w304 -> [w354] mode=indexing
              tunnel: w307 -> [w356]
              tunnel: w308 -> [w349]
              w348 = refnum<vi> refnum  # Node
              w352 = refnum<vi> refnum  # Node
              n147 = To More Specific Class(target class=w352, reference=w354) -> (specific class reference=w353:refnum<vi>)  [unwired: 1 in, 1 out]
              n148 = property class="Node"(reference=w353, error in=w355) -> ("Desc"=w340:string)  [unwired: 2 out]
              n149 = Equal?(x=w340, y="ClassAttribute") -> (x = y?=w351:bool)
              n150 = Compound Arithmetic op=AND(w351, invert w349) -> (w350:bool)
              n151 = Select(t=w356, s=w350, f=w357) -> (s? t:f=w358:path)
              n152 = invoke class="GObj" method="Replace"(reference=w354, error in=w355, "Path"=w358) -> (error out=w342:errorcluster, "Replace"=w347:refnum<vi>)  [unwired: 3 in, 4 out]
              n153 = To More Specific Class(target class=w348, reference=w347, error in=w342) -> (specific class reference=w346:refnum<vi>, error out=w345:errorcluster)
              n154 = property class="Node"(reference=w346, error in=w345, "Desc"=w340) -> (reference out=w343:refnum<vi>, error out=w341:errorcluster)
            }
            n155 = Not(x=w308) -> (.not. x?=w301:bool)
            n156 = Close Reference(reference=w304, error in (no error)=w323) -> (error out=w303:errorcluster)
            n157 = Close Reference(reference=w332, error in (no error)=w323) -> ()  [unwired: 1 out]
            n158 = invoke class="VI" method="BD.Remove Bad Wires"(reference=w324, error in=w323) -> (error out=w322:errorcluster)  [unwired: 1 in, 2 out]
            n159 = Close Reference(reference=w302, error in (no error)=w303) -> ()  [unwired: 1 out]
            n160 = Select(t="EnableDisableStruture", s=w301, f="UpdateIcons") -> (s? t:f=w311:string)
            n161 = Bundle By Name(cluster=w310, "ClassAttribute"=w301) -> (w309:T3)
          }
          frame "EnableDisableStruture" {
            n162 = Unbundle By Name(w360) -> ("Template_GetObjectStatusRef"=w359:refnum<vi>)
            n163 = call <resource>:"Scripting_FindNodeOnDiagram.vi"("ViRef(Ignored If Not Wired)"=w359, "NodeTypesToSearchFor"=string[] ["DisableStructure"], "error in (no error)"=w362) -> ("Nodes"=w366:refnum<vi>[], "error out"=w364:errorcluster)  [unwired: 15 in]
            n164 = for {
              tunnel: w366 -> [w375] mode=indexing
              shift-right: [w368] -> w365
              shift-left: w364 -> [w371]
              w373 = i16 0 ("number")
              w374 = refnum<vi> refnum  # DisableStructure
              n165 = To More Specific Class(target class=w374, reference=w375, error in=w371) -> (specific class reference=w369:refnum<vi>, error out=w370:errorcluster)
              n166 = To Word Integer(number=w373) -> (16bit integer=w372:i16)
              n167 = property class="DisableStructure"(reference=w369, error in=w370, "VisFrame"=w373, "ActiveFrame"=w372) -> (error out=w368:errorcluster)  [unwired: 1 out]
            }
            n168 = Close Reference(reference=w366, error in (no error)=w365) -> (error out=w361:errorcluster)
          }
          frame "UpdateIcons" {
            w409 = u8 32 ("x")
            n169 = Unbundle By Name(w393) -> ("Template_GetObjectStatusRef"=w382:refnum<vi>)
            n170 = property class="LVClassLibrary"(reference=w394, error in=w391) -> (reference out=w399:refnum<vi>, error out=w395:errorcluster, "Member Data"=w397:refnum<vi>)
            n171 = call <resource>:"GDSLvIcon_AnalyseViIcon.vi"("ViRef/LvCLassRef/LvLibRef/ViPath/2D_Image"=w397, "error in (no error)"=w395) -> ("HeaderIcon"=w400:u8[][], "error out"=w396:errorcluster)  [unwired: 5 in, 11 out]
            n172 = Close Reference(reference=w397, error in (no error)=w396) -> (error out=w398:errorcluster)
            n173 = Array Size(array=w400) -> (size(s)=w404:i32[])
            n174 = call <resource>:"GDSLvClass_ReadClassColors.vi"("Library Refnum"=w399, "error in (no error)"=w398) -> ("LvClassIconSettings"=w402:T12, "error out"=w392:errorcluster)  [unwired: 12 in, 4 out]
            n175 = Unbundle By Name(w402) -> ("Frame"=w403:u32, "Frame thickness"=w401:u8)  [unwired: 1 out]
            n176 = Index Array(array=w404) -> (element #1=w406:i32)  [unwired: 2 in, 1 out]
            n177 = Unbundle By Name(w402) -> ("ColorPublic"=w378:u32)
            n178 = Multiply(x=w401, y=u8 2) -> (x*y=w407:u8)
            n179 = Add(x=w406, y=w407) -> (x+y=w408:i32)
            n180 = Increment(x=w408) -> (x+1=w410:i32)
            n181 = call <resource>:"GDSLvIcon_AnalyseViIcon.vi"("ViRef/LvCLassRef/LvLibRef/ViPath/2D_Image"=w382, "error in (no error)"=w392) -> ("BodyIcon"=w381:u8[][], "BodyBkColor"=w376:u32, "error out"=w383:errorcluster)  [unwired: 5 in, 10 out]
            n182 = Subtract(x=w409, y=w410) -> ()  [unwired: 1 out]
            n183 = Subtract(x=w409, y=w407) -> ()  [unwired: 1 out]
            n184 = call <resource>:"GDSLvIcon_Convert24bitTo8bitColor.vi"("Color 24bit In"=w378) -> ("Color out(256)"=w377:u8)  [unwired: 15 in, 3 out]
            n185 = call <resource>:"GDSLvIcon_Convert24bitTo8bitColor.vi"("Color 24bit In"=w376) -> ("Color out(256)"=w379:u8)  [unwired: 15 in, 3 out]
            n186 = for {
              tunnel: w381 -> [w415] mode=indexing
              tunnel: [w414] -> w380 mode=indexing
              tunnel: w377 -> [w413]
              tunnel: w379 -> [w412]
              n187 = for {
                tunnel: w415 -> [w419] mode=indexing
                tunnel: [w418] -> w414 mode=indexing
                tunnel: w413 -> [w417]
                tunnel: w412 -> [w416]
                n188 = Equal?(x=w416, y=w419) -> (x = y?=w420:bool)
                n189 = Select(t=w417, s=w420, f=w419) -> (s? t:f=w418:u8)
              }
            }
            n190 = call <resource>:"GDSLvIcon_CreateIconPicture.vi"("FrameColor"=w403, "FrameThickness(1)"=w401, "HeaderIconIn"=w400, "BodyIconIn"=w380, "error in (no error)"=w383) -> ("WholeIconOut"=w385:u8[][], "error out"=w388:errorcluster)  [unwired: 9 in, 4 out]
            n191 = Reshape Array(w385, 1024 ("dimension size")) -> (w387:u8[])
            n192 = Bundle By Name(cluster=T7 {"image type"=0, "image depth"=8, "image"=[], "mask"=[], "colors"=[], "Rectangle"={"left"=0, "top"=0, "right"=32, "bottom"=32}} ("image data"), "image"=w387) -> (w389:T7)
            n193 = invoke class="VI" method="VI Icon.Set from Image Data"(reference=w382, error in=w388, "ImageData"=w389) -> (error out=w390:errorcluster)  [unwired: 3 in, 5 out]
          }
        }
        n194 = Equal?(x=w114, y="Exit") -> (x = y?=w117:bool)
        n195 = Select(t="Error", s=w113, f=w114) -> (s? t:f=w118:string)
      }
    }
    frame "RemovePattern" {
    }
    frame "CreatePatternMethod" {
    }
  }
  "error out" <- w8
  "DataOut" <- w5
  "Cancelled" <- w6
  "Name" <- "Debugging" ("Name")
